vi "delete emputy column.vi"(11 "input_eeprom":string[][](array[string])) -> (3 "input_eeprom_deleteemputycolumn":string[][](array[string]))   [LabVIEW 2011]
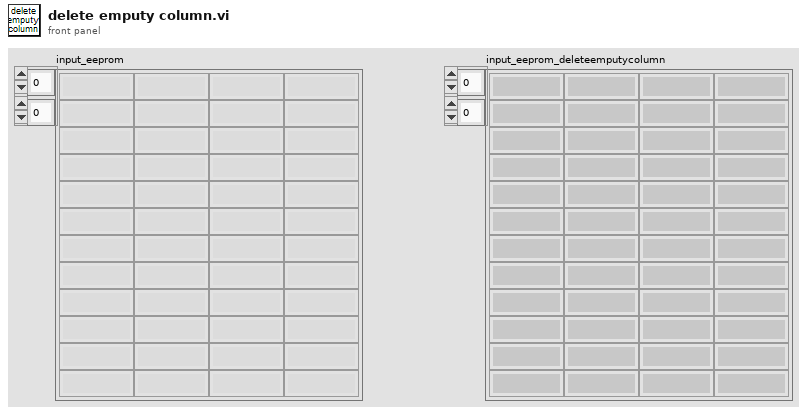
[diagram p1: front panel]
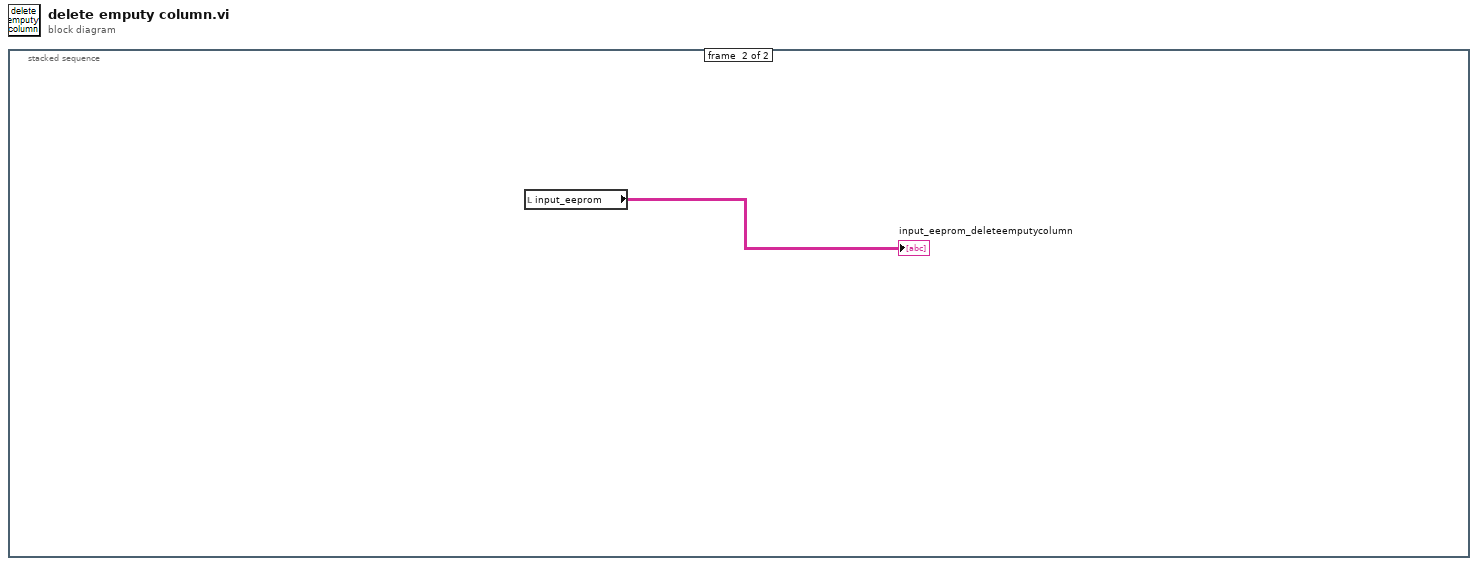
[diagram p0: block diagram]
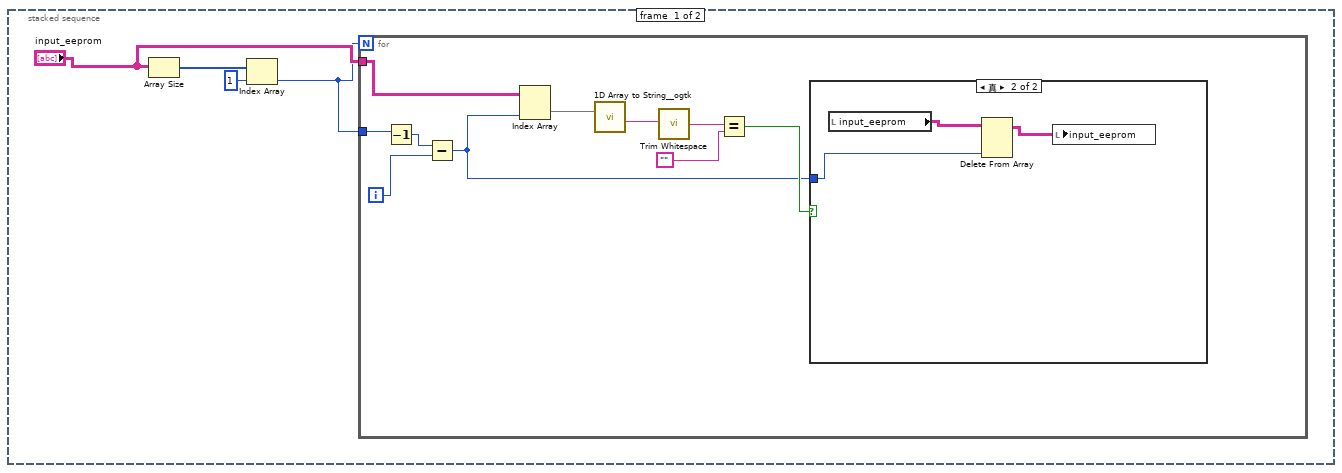
[diagram p2: hidden frame]
diagram:
  n1 = stacked-sequence {
    frame #0 {
      n2 = Array Size(array="input_eeprom") -> (size(s)=w4:i32[])
      n3 = Index Array(array=w4, index=1 ("索引")) -> (element=w1:i32)
      n4 = for {
        N: w1 -> [_]
        tunnel: "input_eeprom" -> [w9]
        tunnel: w1 -> [w7]
        i -> [w8]
        n5 = Decrement(x=w7) -> (x-1=w6:i32)
        n6 = Subtract(x=w6, y=w8) -> (x-y=w5:i32)
        n7 = Index Array(array=w9, index (col)=w5) -> (element=w14:string[])  [unwired: 1 in]
        n8 = call <userlib>:"1D Array to String__ogtk.vi"("Array of Strings"=w14) -> ("delimited string"=w13:string)  [unwired: 10 in]
        n9 = call <vilib>:"Trim Whitespace.vi"("string"=w13) -> ("trimmed string"=w12:string)  [unwired: 1 in]
        n10 = Equal?(x=w12, y="") -> (x = y?=w10:bool)
        n11 = case shown="真" w10 {
          tunnel: w5 -> [_ w16]
          frame False {
          }
          frame True {
            n12 = local read "input_eeprom"() -> (w17:string[][])
            n13 = Delete From Array(array=w17, index (col)=w16) -> (array with subset deleted=w15:string[][])  [unwired: 2 in, 1 out]
            n14 = local write "input_eeprom"(w15) -> ()
          }
        }
      }
    }
    frame #1 {
      n15 = local read "input_eeprom"() -> (→"input_eeprom_deleteemputycolumn":string[][])
    }
  }
